vi "setTiming.vi"(2 "error in (no error)":errorcluster, 3 "HamegHMPSupply in":refnum<class "HamegHMPSupply.lvclass">) -> (0 "error out":errorcluster, 1 "HamegHMPSupply out":refnum<class "HamegHMPSupply.lvclass">)   [LabVIEW 2011, in "Hardware.lvlib" / "Channels.lvlib" / "HamegHMPSupply.lvclass"]
doc: "Abstract Methods.\n\nUse this vi to set the timing and triggering information for the analog output channel."
uses:
  HamegHMPSupply.lvclass
  AnalogOutput.lvclass
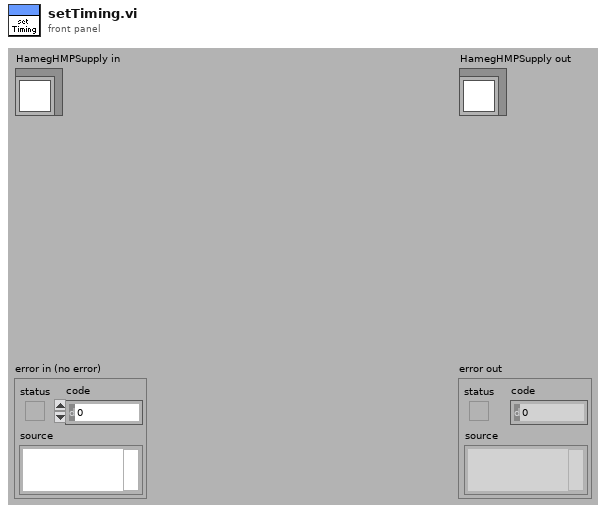
[diagram p1: front panel]
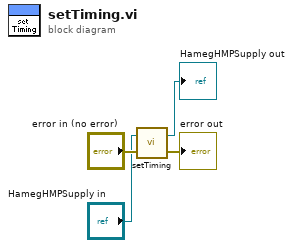
[diagram p0: block diagram]
diagram:
  n1 = call-parent "setTiming.vi"("error in (no error)"="error in (no error)", "AnalogOutput in"="HamegHMPSupply in") -> ("error out"=→"error out":errorcluster, "AnalogOutput out"=→"HamegHMPSupply out":refnum<class "HamegHMPSupply.lvclass">)
